vi "Run Test - Time Stirngs to Seconds (SubVI).vi"(11 "Time String":string[](array[string])) -> (3 "Seconds":sgl[](array[numeric]))   [LabVIEW 2019]
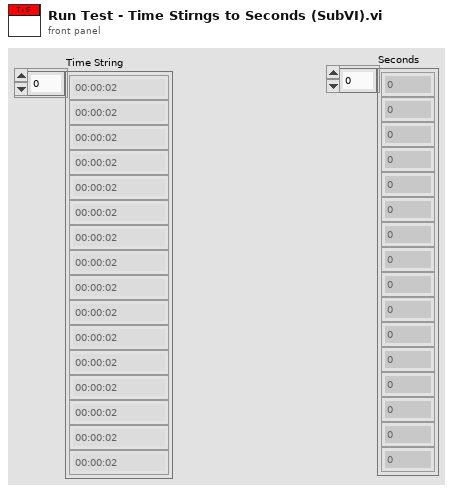
[diagram p1: front panel]
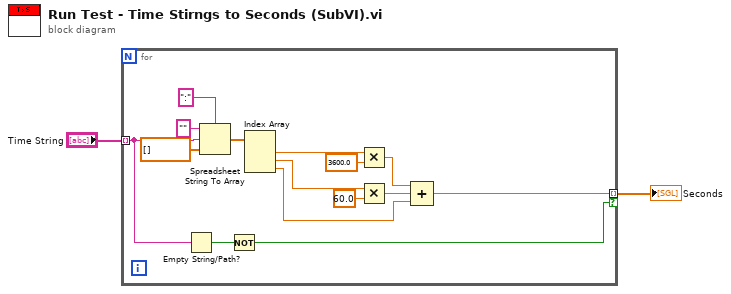
[diagram p0: block diagram]
diagram:
  n1 = for {
    tunnel: "Time String" -> [w5] mode=indexing
    tunnel: [w6] -> w1 mode=indexing if=w3
    n2 = Empty String/Path?(string/path=w5) -> (empty?=w4:bool)
    n3 = Spreadsheet String To Array(delimiter (Tab)=":", format string="", spreadsheet string=w5, array type (2D Dbl)=sgl[] []) -> (array=w14:sgl[])
    n4 = Not(x=w4) -> (.not. x?=w3:bool)
    n5 = Index Array(array=w14) -> (element #1=w9:sgl, element #2=w8:sgl, element #3=w7:sgl)  [unwired: 3 in]
    n6 = Multiply(x=w9, y=sgl 3600.0) -> (x*y=w12:sgl)
    n7 = Multiply(x=w8, y=sgl 60.0) -> (x*y=w13:sgl)
    n8 = Compound Arithmetic op=ADD(w12, w13, w7) -> (w6:sgl)
  }
  "Seconds" <- w1
